vi "GT Get Enc Pos Pre.vi"(6 "pClock":u32, 7 "count":i16, 8 "error in (no error)":errorcluster caption="错误输入（无错误）", 9 "pValue":dbl, 10 "encoder":i16, 11 "cardNum":i16) -> (0 "error out":errorcluster caption="错误输出", 1 "pValue out":dbl, 3 "function return":i16, 4 "pClock out":u32)   [LabVIEW 2020, in "gts.lvlib"]
doc: "GT_API GT_GetEncPosPre(short cardNum,short encoder,double *pValue,short count=1,unsigned long *pClock=NULL);"
uses:
  gts.lvlib
  dll/32bit/multi_card/gts.dll
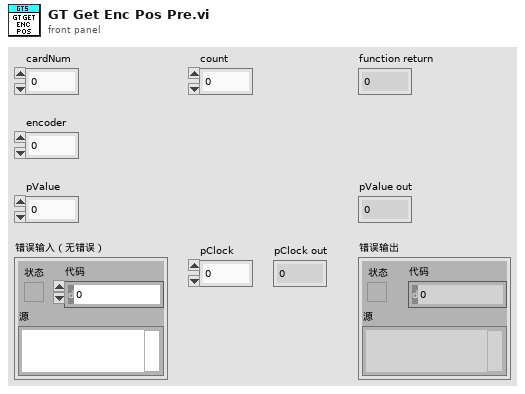
[diagram p1: front panel]
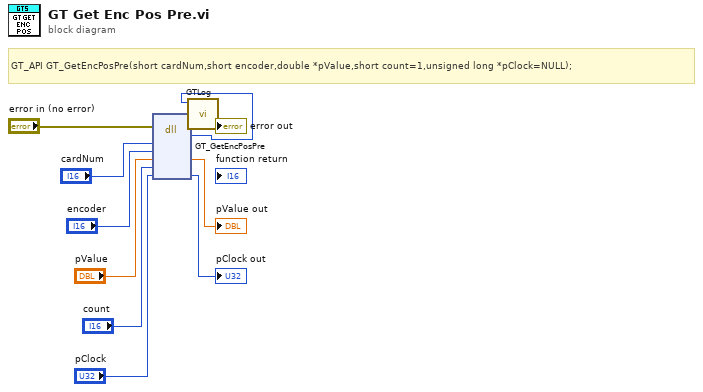
[diagram p0: block diagram]
diagram:
  # "GT_API GT_GetEncPosPre(short cardNum,short encoder,double *pValue,short count=1,unsigned long *pClock=NULL);"
  n1 = dll-call lib="C:/1228/dll/32bit/multi_card/gts.dll" fn="GT_GetEncPosPre"(error in="error in (no error)", "cardNum"="cardNum", "encoder"="encoder", "pValue"="pValue", "count"="count", "pClock"="pClock") -> (error out=w3:errorcluster, w1:i16, "pValue"=→"pValue out":dbl, "pClock"=→"pClock out":u32)  [unwired: 5 in, 1 out]
  n2 = call "GTLog.vi"("error in (no error)"=w3, "Numeric"=w1) -> ("error out"=→"error out":errorcluster)  [unwired: 9 in]
